vi "VI Dynamic Call.vi"(6 "FP State":T2={"Activate?"=TRUE, "State"=enum."Minimized"}, 8 "error in (no error)":errorcluster, 9 "Control Values":T1(array[cluster]), 10 "VI Name":string="Dynamic Buffer Handler.vi", 11 "Parent Path":path) -> (0 "error out":errorcluster, 2 "Clone Name":string, 3 "reference out":refnum<vi>)   [LabVIEW 2019]
panel:
  out "appended path":path
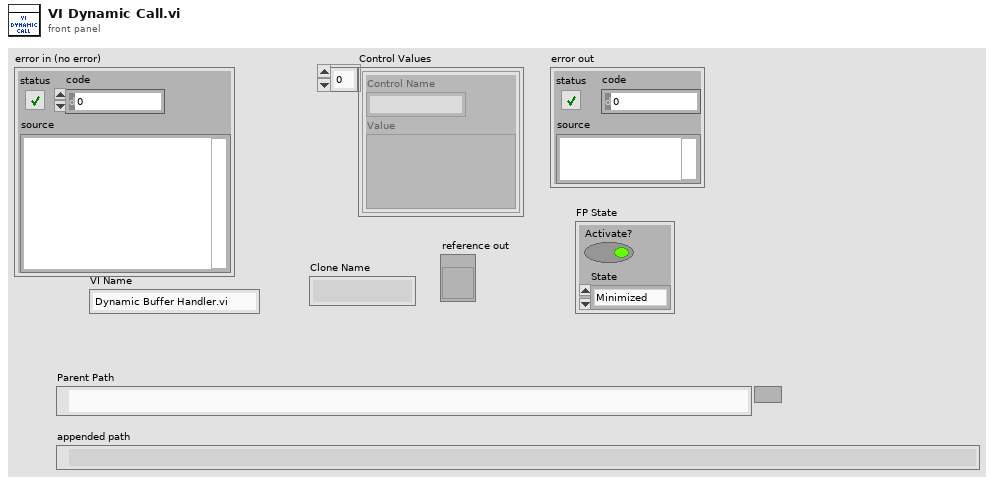
[diagram p1: front panel]
types:
  T1 = cluster{"Control Name":string, "Value":variant}[]
  T2 = cluster{"Activate?":bool, "State":enum32{"Invalid", "Standard", "Closed", "Hidden", "Minimized", "Maximized"}}
  T3 = enum32{"Invalid", "Standard", "Closed", "Hidden", "Minimized", "Maximized"}
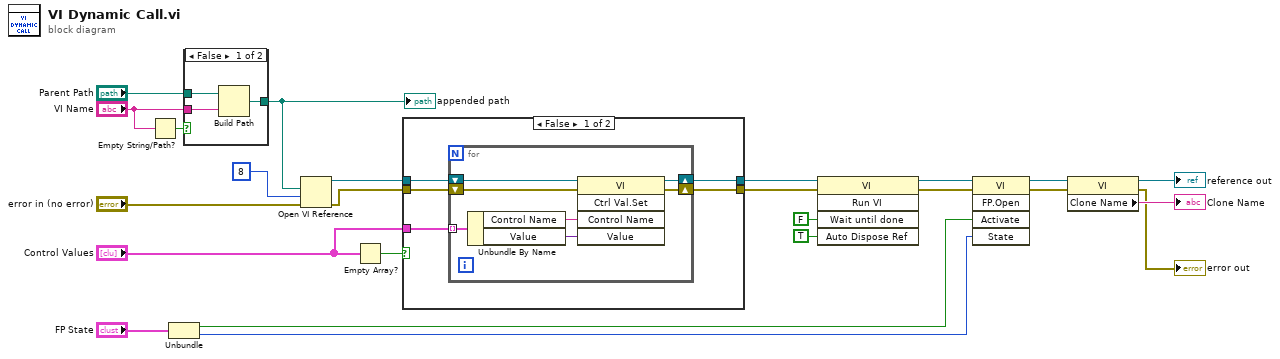
[diagram p0: block diagram]
diagram:
  n1 = Empty String/Path?(string/path="VI Name") -> (empty?=w1:bool)
  n2 = Unbundle("FP State") -> ("Activate?"=w13:bool, "State"=w12:T3)
  n3 = case shown="False" w1 {
    tunnel: [w27 w28] -> w20
    tunnel: "VI Name" -> [w26 _]
    tunnel: "Parent Path" -> [w25 w28]
    frame False {
      n4 = Build Path(base path=w25, name or relative path=w26) -> (appended path=w27:path)
    }
    frame True {
    }
  }
  "appended path" <- w20
  n5 = Open VI Reference(vi path=w20, options=8, error in (no error)="error in (no error)") -> (vi reference=w7:refnum<vi>, error out=w6:errorcluster)  [unwired: 3 in]
  n6 = Empty Array?(array="Control Values") -> (empty?=w10:bool)
  n7 = case shown="False" w10 {
    tunnel: w7 -> [w33 w42]
    tunnel: [w32 w42] -> w9
    tunnel: w6 -> [w31 w41]
    tunnel: [w29 w41] -> w8
    tunnel: "Control Values" -> [w30 _]
    frame False {
      n8 = for {
        shift-right: [w39] -> w32
        shift-left: w33 -> [w40]
        shift-right: [w37] -> w29
        shift-left: w31 -> [w38]
        tunnel: w30 -> [w36] mode=indexing
        n9 = Unbundle By Name(w36) -> ("Control Name"=w35:string, "Value"=w34:variant)
        n10 = invoke class="VI" method="Ctrl Val.Set"(reference=w40, error in=w38, "Control Name"=w35, "Value"=w34) -> (reference out=w39:refnum<vi>, error out=w37:errorcluster)  [unwired: 1 in, 3 out]
      }
    }
    frame True {
    }
  }
  n11 = invoke class="VI" method="Run VI"(reference=w9, error in=w8, "Wait until done"=FALSE ("Wait Until Done"), "Auto Dispose Ref"=TRUE ("Auto Dispose Reference")) -> (reference out=w17:refnum<vi>, error out=w16:errorcluster)  [unwired: 1 in, 3 out]
  n12 = invoke class="VI" method="FP.Open"(reference=w17, error in=w16, "Activate"=w13, "State"=w12) -> (reference out=w5:refnum<vi>, error out=w4:errorcluster)  [unwired: 1 in, 3 out]
  n13 = property class="VI"(reference=w5, error in=w4) -> (reference out=→"reference out":refnum<vi>, error out=→"error out":errorcluster, "Clone Name"=→"Clone Name":string)
